vi "C843_Sample_Application_2a.vi"() -> ()   [LabVIEW 2015]
doc: "This VI demonstrates how to statically define a C-843 configuration with two C-843 2-channel boards and connected stages. In this \nexample, stage M-405.PD is attached to axis one and two of both boards. The VI runs C843_Configuration_Setup.vi for both boards\nwith these pre-defined settings and reads the position of all axes. The diagram shows how to combine the driver VIs for these tasks. \n\nWarning: This VI has stages defined for each axis that probably do not match your current configuration. Please modify the \"Stages \nnames input\" array in the diagram before running the VI."
panel:
  in  "stop":bool
  out "Position system 2":dbl[](array[numeric]) format="%.6f"
  out "Identification board 2":string
  out "Conn. Axes board 2":string[](array[string])
  in  "error in":errorcluster
  out "Running":bool caption="Axes are referencing"
  out "error out":errorcluster
  out "Position system 1":dbl[](array[numeric]) format="%.6f"
  out "Conn. Axes board 1":string[](array[string])
  out "Identification board 1":string
  # "Simple C-843 sample program"
  # "This VI demonstrates how to statically define a C-843 configuration with two C-843 2-channel boards and connected stages. In this \nexample, stage M-405.PD is attached to axis one and two of both boards. The VI runs C843_Configuration_Setup.vi for both boards\nwith these pre-defined settings and reads the position of all axes. The diagram shows how to combine the driver VIs for these tasks. \n\nWarning: This VI has stages defined for each axis that probably do not match your current configuration. Please modify the \"Stages \nnames input\" array in the diagram before running the VI."
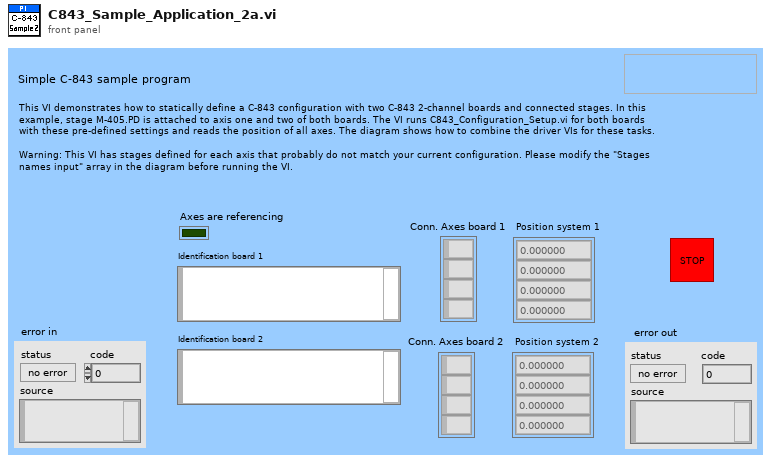
[diagram p1: front panel]
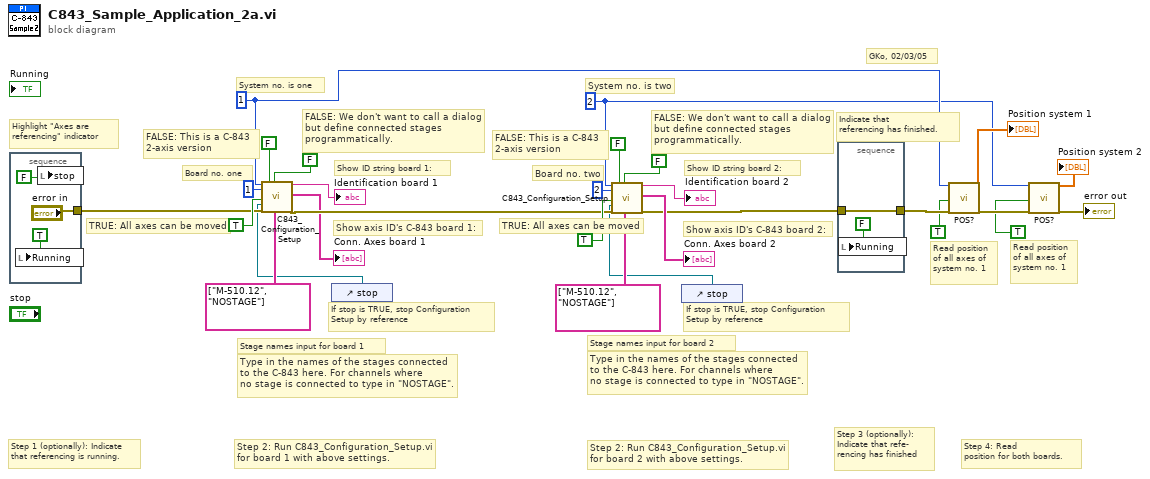
[diagram p0: block diagram]
diagram:
  w2 = 2 ("System no.")
  w3 = 1 ("System no.")
  # "Read position\nof all axes of\nsystem no. 1"
  # "Read position\nof all axes of\nsystem no. 1"
  # "If stop is TRUE, stop Configuration\nSetup by reference"
  # "If stop is TRUE, stop Configuration\nSetup by reference"
  # "Step 2: Run C843_Configuration_Setup.vi\nfor board 2 with above settings."
  # "Type in the names of the stages connected\nto the C-843 here. For channels where\nno stage is connected to type in \"NOSTAGE\"."
  # "Stage names input for board 2"
  # "Show axis ID's C-843 board 2:"
  # "Show ID string board 2:"
  # "FALSE: We don't want to call a dialog\nbut define connected stages\nprogrammatically."
  # "TRUE: All axes can be moved"
  # "Board no. two"
  # "System no. is two"
  # "FALSE: This is a C-843 \n2-axis version"
  # "Stage names input for board 1"
  # "GKo, 02/03/05"
  # "Step 4: Read \nposition for both boards."
  # "Step 3 (optionally): \nIndicate that refe-\nrencing has finished"
  # "Step 2: Run C843_Configuration_Setup.vi\nfor board 1 with above settings."
  # "Step 1 (optionally): Indicate\nthat referencing is running."
  # "Indicate that\nreferencing has finished."
  # "Highlight \"Axes are\nreferencing\" indicator"
  # "Show axis ID's C-843 board 1:"
  # "Show ID string board 1:"
  # "FALSE: We don't want to call a dialog\nbut define connected stages\nprogrammatically."
  # "Type in the names of the stages connected\nto the C-843 here. For channels where\nno stage is connected to type in \"NOSTAGE\"."
  # "TRUE: All axes can be moved"
  # "Board no. one"
  # "System no. is one"
  # "FALSE: This is a C-843 \n2-axis version"
  n1 = stacked-sequence {
    tunnel: ["error in"] -> w22
    frame #0 {
      n2 = local write "Running"(TRUE ("Running")) -> ()
      n3 = local write "stop"(FALSE ("stop")) -> ()
    }
  }
  n4 = control-ref of="stop"() -> (w5:refnum<vi>)
  n5 = call "C843_Configuration_Setup.vi"("System no."=w3, "C-843 Board No."=1, "All axes?"=TRUE, "Stop refnum"=w5, "error in"=w22, "C-843 version"=FALSE, "Use dialog to define\nconnected stages?"=FALSE ("Use dialog to define\nconnected stages?"), "Stage names input"=string[] ["M-510.12", "NOSTAGE"]) -> ("Identification"=→"Identification board 1":string, "Conn. \nAxes"=→"Conn. Axes board 1":string[], "error out"=w14:errorcluster)  [unwired: 7 in, 2 out]
  n6 = control-ref of="stop"() -> (w4:refnum<vi>)
  n7 = call "C843_Configuration_Setup.vi"("System no."=w2, "C-843 Board No."=2, "All axes?"=TRUE, "Stop refnum"=w4, "error in"=w14, "C-843 version"=FALSE, "Use dialog to define\nconnected stages?"=FALSE ("Use dialog to define\nconnected stages?"), "Stage names input"=string[] ["M-510.12", "NOSTAGE"]) -> ("Identification"=→"Identification board 2":string, "Conn. \nAxes"=→"Conn. Axes board 2":string[], "error out"=w13:errorcluster)  [unwired: 7 in, 2 out]
  n8 = stacked-sequence {
    tunnel: w13 -> [w33]
    tunnel: [w33] -> w12
    frame #0 {
      n9 = local write "Running"(FALSE ("Running")) -> ()
    }
  }
  n10 = call "POS?.vi"("System no."=w3, "All axes?"=TRUE, "error in"=w12) -> ("Position"=→"Position system 1":dbl[], "error out"=w11:errorcluster)  [unwired: 2 in, 13 out]
  n11 = call "POS?.vi"("System no."=w2, "All axes?"=TRUE, "error in"=w11) -> ("Position"=→"Position system 2":dbl[], "error out"=→"error out":errorcluster)  [unwired: 2 in, 13 out]
